vi "Test Skip Test.vi"(8 "error in (no error)":errorcluster, 11 "LUnit Test Case V2 Test Double In":refnum<class "LUnit Test Case V2 Test Double.lvclass">) -> (0 "error out":errorcluster, 3 "LUnit Test Case V2 Test Double Out":refnum<class "LUnit Test Case V2 Test Double.lvclass">)   [LabVIEW 2020, in "LUnit Test Case V2 Test Double.lvclass"]
uses:
  LUnit Test Case V2 Test Double.lvclass
  C:/Git/astemes-lunit/source/Rewrite Project/LUnit Test Case/LUnit Test Case V2.lvclass
  LUnit Test Case/LUnit Test Case V2.lvclass/LUnit Test Case V2.ctl
  LUnit Test Case V2 Test Double.lvclass/LUnit Test Case V2 Test Double.ctl
  LUnit Test Case/LUnit Test Case V2.lvclass
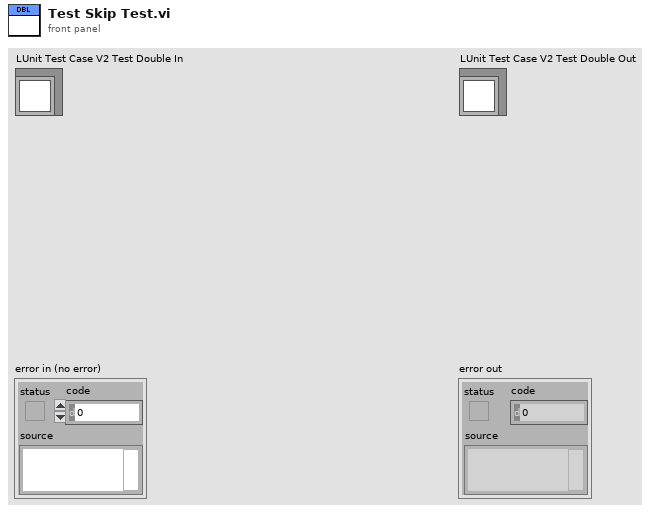
[diagram p1: front panel]
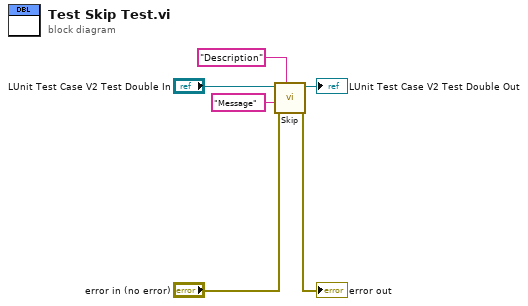
[diagram p0: block diagram]
diagram:
  n1 = call "Skip.vi"("Description"="Description", "error in (no error)"="error in (no error)", "Message"="Message", "LUnit Test Case In"="LUnit Test Case V2 Test Double In") -> ("error out"=→"error out":errorcluster, "LUnit Test Case Out"=→"LUnit Test Case V2 Test Double Out":refnum<class "LUnit Test Case V2 Test Double.lvclass">)  [unwired: 6 in]
